vi "get_all_switches.vi"(8 "error in (no error)":errorcluster, 11 "Agilent 34980A in":refnum<class "Agilent 34980A.lvclass">) -> (0 "error out":errorcluster, 2 "actual switch states":bool[](array[boolean]), 3 "Agilent 34980A out":refnum<class "Agilent 34980A.lvclass">)   [LabVIEW 2018, in "Agilent 34980A.lvclass"]
doc: "gets/reads the actual state of the switches from the instrument"
uses:
  Agilent 34980A.lvclass
  instrument.lvclass
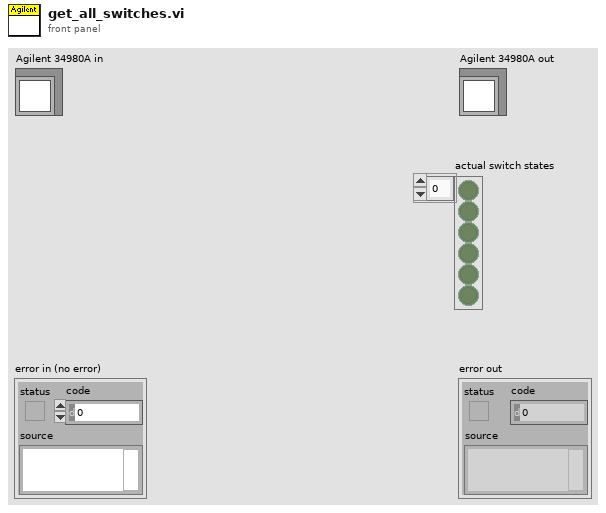
[diagram p1: front panel]
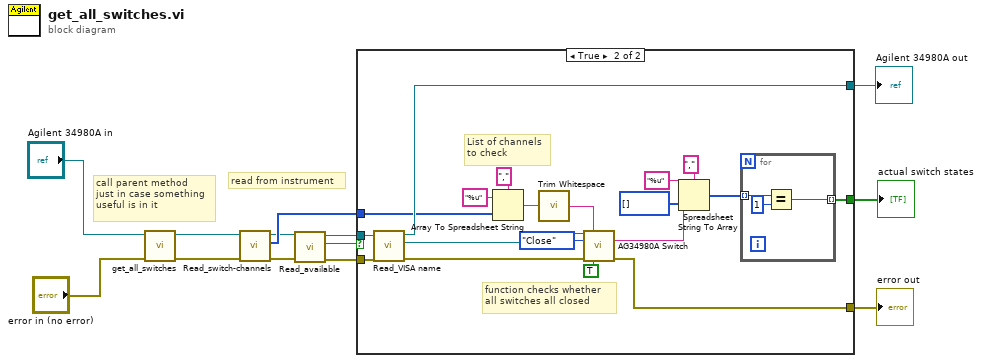
[diagram p0: block diagram]
diagram:
  # "read from instrument"
  # "call parent method \njust in case something\nuseful is in it"
  n1 = call-parent "get_all_switches.vi"("error in (no error)"="error in (no error)", "instrument in"="Agilent 34980A in") -> ("error out"=w8:errorcluster, "instrument out"=w9:refnum<class "Agilent 34980A.lvclass">)  [unwired: 7 in, 1 out]
  n2 = call-dynamic "Read_switch-channels.vi"("error in (no error)"=w8, "instrument in"=w9) -> ("error out"=w3:errorcluster, "switch channels"=w7:u16[], "instrument out"=w5:refnum<class "Agilent 34980A.lvclass">)  [unwired: 7 in]
  n3 = call-dynamic "Read_available.vi"("error in (no error)"=w3, "instrument in"=w5) -> ("error out"=w2:errorcluster, "available?"=w1:bool, "instrument out"=w4:refnum<class "Agilent 34980A.lvclass">)  [unwired: 7 in]
  n4 = case shown="True" w1 {
    tunnel: [w15 w32] -> w11
    tunnel: [w14 w30] -> w10
    tunnel: w7 -> [_ w28]
    tunnel: [_ w18] -> w6
    tunnel: w4 -> [w15 w17]
    tunnel: w2 -> [w14 w16]
    frame False {
    }
    frame True {
      # "function checks whether\nall switches all closed"
      # "List of channels\nto check"
      n5 = call-dynamic "Read_VISA name.vi"("error in (no error)"=w16, "instrument in"=w17) -> ("error out"=w31:errorcluster, "VISA resource name"=w34:refnum<visa-resource-name>, "instrument out"=w32:refnum<class "Agilent 34980A.lvclass">)  [unwired: 7 in]
      n6 = Array To Spreadsheet String(delimiter (Tab)=",", array=w28, 3:"%u" ("format string")) -> (spreadsheet string=w25:string)
      n7 = call <vilib>:"Trim Whitespace.vi"("string"=w25) -> ("trimmed string"=w24:string)  [unwired: 1 in]
      n8 = call "AG34980A Switch.vi"("VISA resource name"=w34, "Channel List"=w24, "Open/Close (0:Close)"=enum16{"Close", "Open"}."Close", "error in (no error)"=w31, "Set/Check (F:Set)"=TRUE) -> ("Channel State?"=w23:string, "error out"=w30:errorcluster)  [unwired: 8 in, 1 out]
      n9 = Spreadsheet String To Array(delimiter (Tab)=",", format string="%u", spreadsheet string=w23, array type (2D Dbl)=u16[] []) -> (array=w19:u16[])
      n10 = for {
        tunnel: w19 -> [w37] mode=indexing
        tunnel: [w35] -> w18 mode=indexing
        n11 = Equal?(x=w37, y=u16 1) -> (x = y?=w35:bool)
      }
    }
  }
  "error out" <- w10
  "Agilent 34980A out" <- w11
  "actual switch states" <- w6
